vi "acquire_image.vi"() -> ()   [LabVIEW 2015, in "camera.lvlib"]
uses:
  camera.lvlib
  Global.vi
  oskar_tools/oskar_tools.lvlib
panel:
  in  "stop":bool
  in  "Tab Control":enum32{"Camera", "Settings"}(tab)
  in  "Pause":bool
  out "Image":T1(plugin-control)
  in  "Zoom":bool
  out "image":i32=22
  in  "max":i32=35000
  in  "min":i32=-35000
  out "Saving":bool
  in  "Exposure (ms)":i32=1000
  in  "Colour":u32(ring) items=["Grayscale", "Binary", "Gradient", "Rainbow", "Temperature", "User Defined"]
  out "Image Pixels (I16)":i16[][](array[numeric])
  out "error out":errorcluster
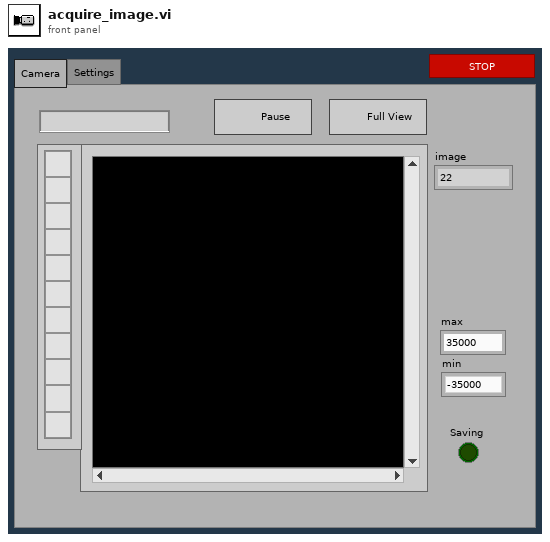
[diagram p1: front panel]
types:
  T1 = typedef "IMAQ Image.ctl" = refnum<image>
  T2 = typedef "Image Type" = u32
  T3 = cluster{"Exposure (ms)":i32, "Manufacturer":string, "Model":string}
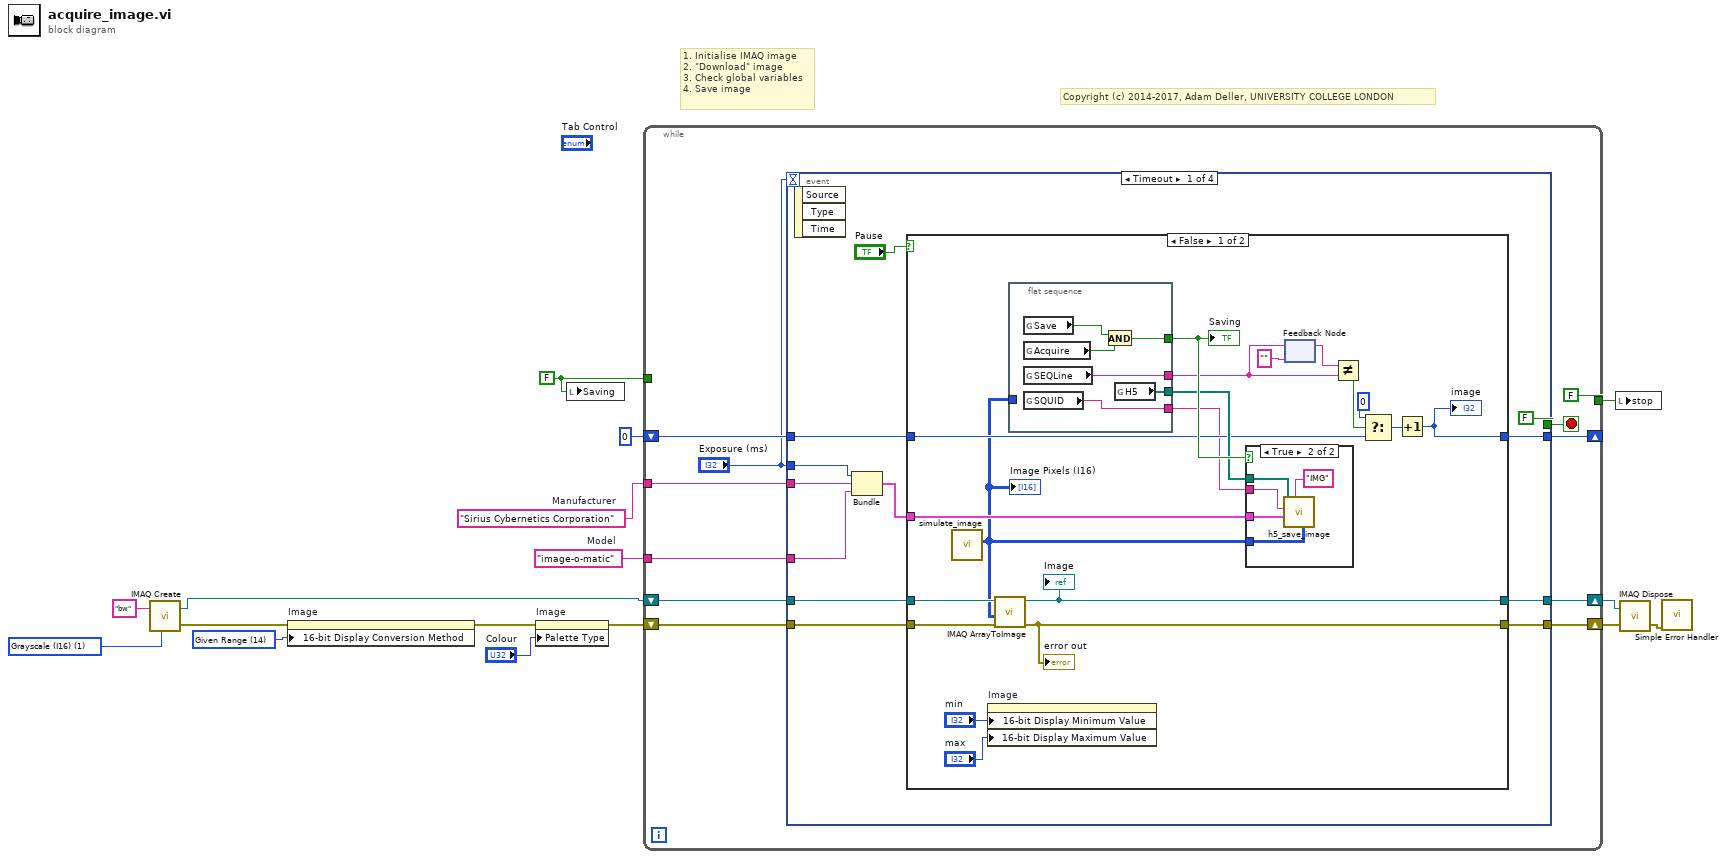
[diagram p0: block diagram]
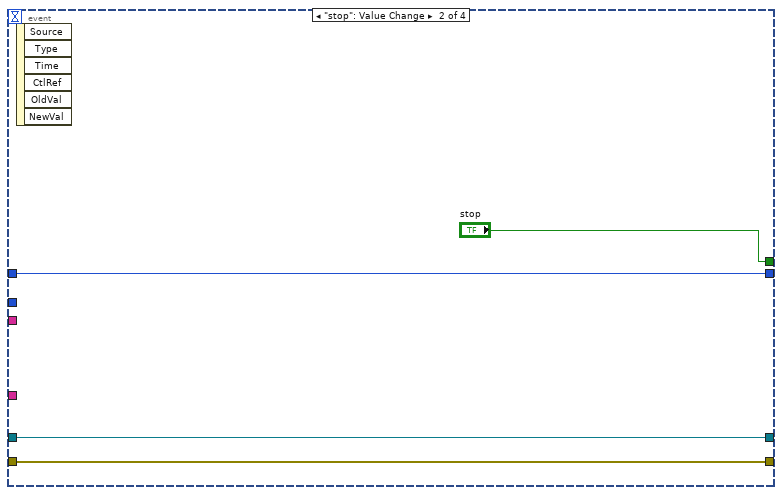
[diagram p4: hidden frame]
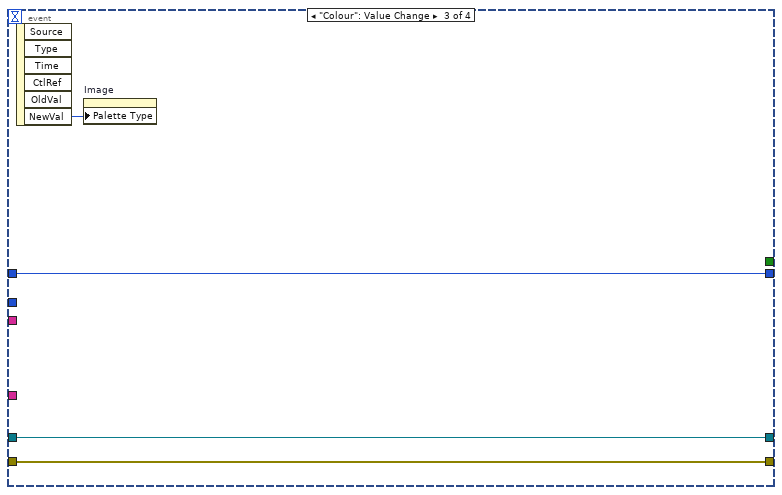
[diagram p5: hidden frame]
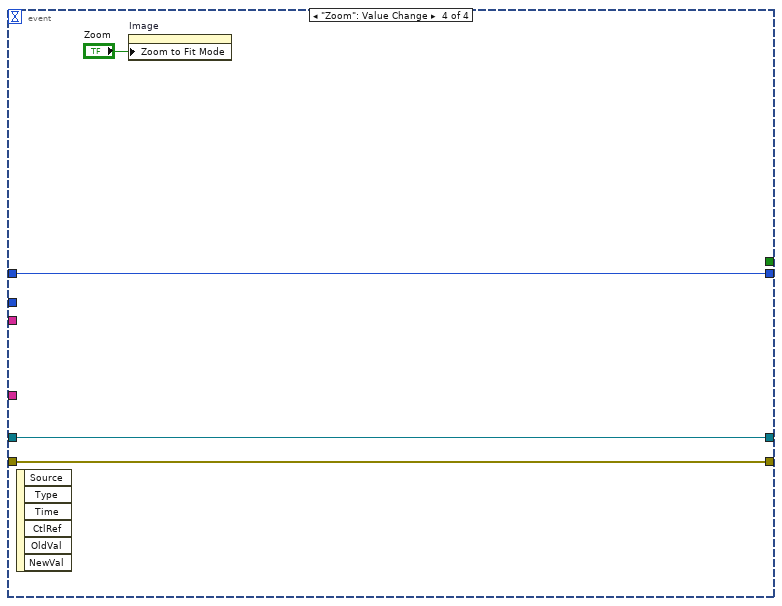
[diagram p6: hidden frame]
diagram:
  w1 = "image-o-matic"  # Model
  w2 = "Sirius Cybernetics Corporation"  # Manufacturer
  w3 = FALSE ("Saving")
  w14 = u32 14 items=["Default"=10, "Most Significant Bits"=11, "Full Dynamic"=12, "Downshift"=13, "Given Range"=14, "90% Dynamic"=15, "Given Percent Range"=16] ("16-bit Display Mapping:Conversion Method")
  w16 = T2 1 items=["Grayscale (U8)", "Grayscale (I16)", "Grayscale (SGL)", "Complex (CSG)", "RGB (U32)", "HSL (U32)", "RGB (U64)", "Grayscale (U16)"] ("Image Type")
  # "1. Initialise IMAQ image\n2. \"Download\" image\n3. Check global variables\n4. Save image"
  # "Copyright (c) 2014-2017, Adam Deller, UNIVERSITY COLLEGE LONDON"
  n1 = call "IMAQ Create"("Image Name"="bw", "Image Type"=w16) -> ("New Image"=w7:T1, "error out"=w6:errorcluster)  [unwired: 3 in]
  n2 = property on="Image" class="ImageControl"(error in=w6, "16-bit Display Conversion Method"=w14) -> (error out=w11:errorcluster)  [unwired: 1 in, 1 out]
  n3 = property on="Image" class="ImageControl"(error in=w11, "Palette Type"="Colour") -> (error out=w5:errorcluster)  [unwired: 1 in, 1 out]
  n4 = local write "Saving"(w3) -> ()
  n5 = while {
    shift-right: [w27] -> w8
    shift-left: w7 -> [w25]
    shift-right: [w24] -> w4
    shift-left: w5 -> [w23]
    shift-right: [w21] -> _
    shift-left: 0 ("Timeout (ms) 2") -> [w22]
    tunnel: [FALSE ("stop")] -> w9
    tunnel: w3 -> [_]
    tunnel: w2 -> [w18]
    tunnel: w1 -> [w17]
    stop <- w26 stop-if-true
    n6 = event shown="[0] Timeout" {
      selector: _ -> [_ _ _ _]
      dyn-events: _ -> [_ _ _ _]
      timeout: "Exposure (ms)" -> [_ _ _ _]
      tunnel: w25 -> [w39 w75 w78 w83]
      tunnel: [w37 w75 w78 w83] -> w27
      tunnel: [FALSE ("Stop") "stop" _ _] -> w26
      tunnel: [w36 w76 w79 w82] -> w24
      tunnel: w23 -> [w38 w76 w79 w82]
      tunnel: w22 -> [w35 w74 w77 w81]
      tunnel: [w34 w74 w77 w81] -> w21
      tunnel: "Exposure (ms)" -> [w30 _ _ _]
      tunnel: w18 -> [w31 _ _ _]
      tunnel: w17 -> [w29 _ _ _]
      event Timeout {
        n7 = event-data() -> ()  [unwired: 1 in, 3 out]
        n8 = Bundle("Exposure (ms)"=w30, "Manufacturer"=w31, "Model"=w29) -> (w28:T3)  [unwired: 1 in]
        n9 = case shown="False" "Pause" {
          tunnel: w39 -> [w48 w72]
          tunnel: w38 -> [w49 w71]
          tunnel: [w47 w72] -> w37
          tunnel: [w46 w71] -> w36
          tunnel: w35 -> [w53 w70]
          tunnel: [w41 w70] -> w34
          tunnel: w28 -> [w43 _]
          frame False {
            n10 = call "simulate_image.vi"() -> ("array"=w40:i16[][])  [unwired: 11 in]
            "Image Pixels (I16)" <- w40
            n11 = property on="Image" class="ImageControl"("16-bit Display Minimum Value"="min", "16-bit Display Maximum Value"="max") -> ()  [unwired: 2 in, 2 out]
            n12 = call "IMAQ ArrayToImage"("error in (no error)"=w49, "Image Pixels (I16)"=w40, "Image"=w48) -> ("error out"=w46:errorcluster, "Image Out"=w47:T1)  [unwired: 7 in]
            "Image" <- w47
            "error out" <- w46
            n13 = flat-sequence {
              tunnel: [w64] -> w56
              tunnel: [w62] -> w54
              tunnel: [w63] -> w55
              tunnel: [w61] -> w50
              tunnel: w40 -> [_]
              frame #0 {
                n14 = global read "Global.vi" "Save"() -> (w60:bool)
                n15 = global read "Global.vi" "Acquire"() -> (w59:bool)
                n16 = global read "Global.vi" "SEQLine"() -> (w62:string)
                n17 = global read "Global.vi" "SQUID"() -> (w61:string)
                n18 = And(x=w60, y=w59) -> (x .and. y?=w64:bool)
                n19 = global read "Global.vi" "H5"() -> (w63:path[])
              }
            }
            n20 = case shown="True" w56 {
              tunnel: w55 -> [_ w66]
              tunnel: w50 -> [_ w67]
              tunnel: w40 -> [_ w69]
              tunnel: w43 -> [_ w68]
              frame False {
              }
              frame True {
                n21 = call "h5_save_image.vi"("array"=w69, "TYPE"="IMG", "Attributes"=w68, "SQUID"=w67, "H5"=w66) -> ()  [unwired: 6 in, 1 out]
              }
            }
            n22 = feedback #1("" ("Seq")) -> (w57:string)
            n23 = feedback-in #1(w54) -> ()
            n24 = Not Equal?(x=w57, y=w54) -> (x != y?=w51:bool)
            n25 = Select(t=0 ("Timeout (ms) 2"), s=w51, f=w53) -> (s? t:f=w42:i32)
            n26 = Increment(x=w42) -> (x+1=w41:i32)
            "image" <- w41
            "Saving" <- w56
          }
          frame True {
          }
        }
      }
      event "stop": Value Change {
        n27 = event-data() -> ()  [unwired: 1 in, 6 out]
      }
      event "Colour": Value Change {
        n28 = event-data() -> ("NewVal"=w80:u32)  [unwired: 1 in, 5 out]
        n29 = property on="Image" class="ImageControl"("Palette Type"=w80) -> ()  [unwired: 2 in, 2 out]
      }
      event "Zoom": Value Change {
        n30 = event-data() -> ()  [unwired: 1 in, 6 out]
        n31 = property on="Image" class="ImageControl"("Zoom to Fit Mode"="Zoom") -> ()  [unwired: 2 in, 2 out]
      }
    }
  }
  n32 = local write "stop"(w9) -> ()
  n33 = call "IMAQ Dispose"("Image"=w8, "error in (no error)"=w4) -> ("error out"=w13:errorcluster)  [unwired: 4 in]
  n34 = call <vilib>:"Simple Error Handler.vi"("error in (no error)"=w13) -> ()  [unwired: 4 in, 5 out]
